vi "Close.vi"(8 "error in":errorcluster, 11 "Capabilities in":refnum<class "Capabilities.lvclass">) -> (0 "error out":errorcluster, 3 "Capabilities out":refnum<class "Capabilities.lvclass">)   [LabVIEW 2023, in "Capabilities.lvclass"]
uses:
  Capabilities.lvclass
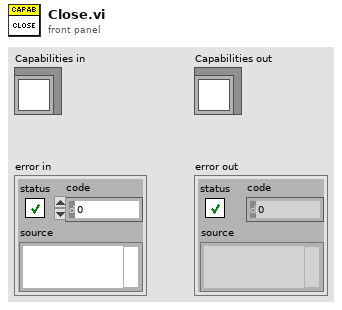
[diagram p1: front panel]
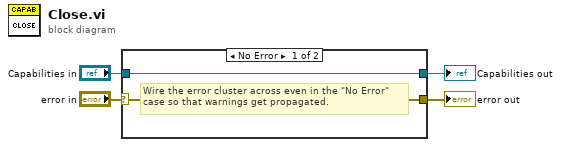
[diagram p0: block diagram]
diagram:
  n1 = case shown="No Error" "error in" {
    selector: "error in" -> [w5 w8]
    tunnel: [w5 w8] -> w1
    tunnel: [w6 w7] -> w3
    tunnel: "Capabilities in" -> [w6 w7]
    frame No Error {
      # "Wire the error cluster across even in the \"No Error\"\ncase so that warnings get propagated."
    }
    frame Error {
    }
  }
  "error out" <- w1
  "Capabilities out" <- w3
